vi "CIVITA_DMARS_conv_PXI(SubVI).vi"(8 "Initial Euler Angles [rad]":cluster{"phi":dbl, "theta":dbl, "psi":dbl}={"phi"=0.766, "theta"=0.643, "psi"=0.0}, 10 "SIM_start":bool, 11 "Civitanav readings [deg]":sgl[](array[numeric])) -> (2 "psi [deg]":dbl, 3 "Euler Angles [rad]":cluster{"phi":dbl, "theta":dbl, "psi":dbl}, 5 "theta [deg]":dbl, 7 "phi [deg]":dbl)   [LabVIEW 2017]
uses:
  <vilib>/Analysis/coordinate.llb/Euler Rotation Order.ctl
  <vilib>/Analysis/baseanly.llb/Real A x B.vi
  <vilib>/Analysis/Matrix/Numeric/Conversions/Array To Matrix - RA2.vi
  <vilib>/Analysis/Matrix/Numeric/Conversions/Matrix To Array - RM.vi
  <vilib>/Analysis/NI_AALPro.lvlib
  <vilib>/Analysis/NI_AALBase.lvlib
  <vilib>/Analysis/Matrix/NI_Matrix.lvlib
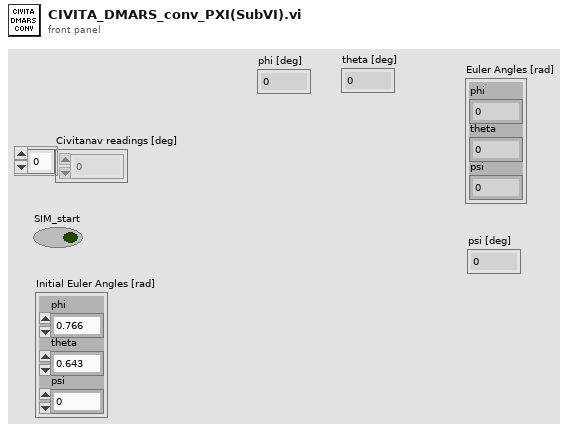
[diagram p1: front panel]
types:
  T1 = typedef "NI_AALPro.lvlib/Euler Rotation Order.ctl" = u16
  T2 = typedef "NI_Matrix.lvlib/RealMatrix.ctl" = dbl[][]
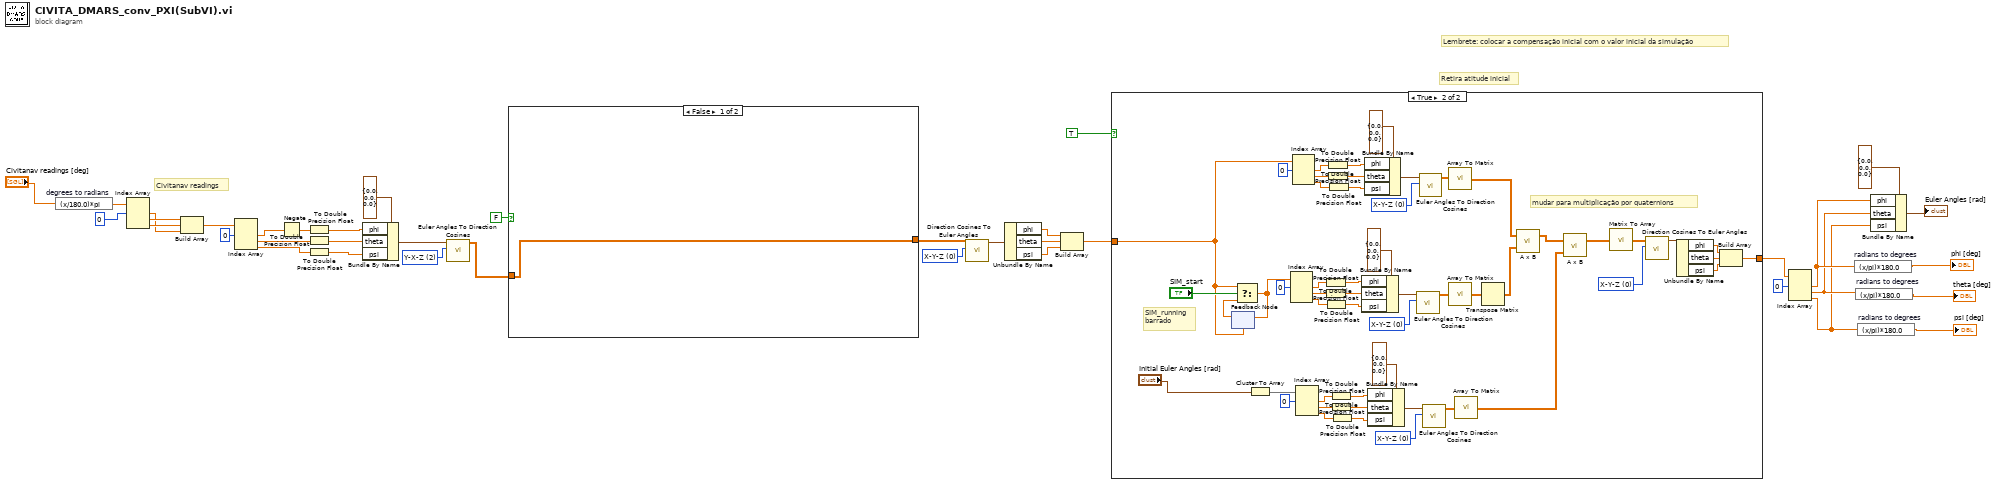
[diagram p0: block diagram]
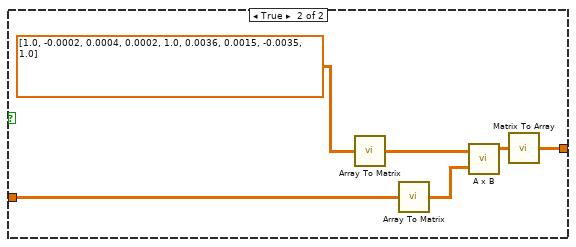
[diagram p3: hidden frame]
diagram:
  w36 = T1 0 items=["X-Y-Z", "X-Z-Y", "Y-X-Z", "Y-Z-X", "Z-X-Y", "Z-Y-X", "X-Y-X", "X-Z-X", "Y-X-Y", "Y-Z-Y", "Z-X-Z", "Z-Y-Z"] ("rotation order")
  w37 = T1 2 items=["X-Y-Z", "X-Z-Y", "Y-X-Z", "Y-Z-X", "Z-X-Y", "Z-Y-X", "X-Y-X", "X-Z-X", "Y-X-Y", "Y-Z-Y", "Z-X-Z", "Z-Y-Z"] ("rotation order")
  # "Lembrete: colocar a compensação inicial com o valor inicial da simulação"
  # "Retira atitude inicial"
  # "Civitanav readings"
  n1 = expression code="(x/180.0)*pi" "degrees to radians"("Civitanav readings [deg]") -> (w31:sgl[])
  n2 = Index Array(array=w31, index #1=0 ("index")) -> (element #1=w27:sgl, element #2=w29:sgl, element #3=w28:sgl)  [unwired: 2 in]
  n3 = Build Array(w29, w28, w27) -> (w17:sgl[])
  n4 = Index Array(array=w17, index #1=0 ("index")) -> (element #1=w23:sgl, element #2=w21:sgl, element #3=w20:sgl)  [unwired: 2 in]
  n5 = Negate(x=w23) -> (-x=w22:sgl)
  n6 = To Double Precision Float(number=w22) -> (double precision float=w3:dbl)
  n7 = To Double Precision Float(number=w21) -> (double precision float=w1:dbl)
  n8 = To Double Precision Float(number=w20) -> (double precision float=w2:dbl)
  n9 = Bundle By Name(cluster=cluster{"phi":dbl, "theta":dbl, "psi":dbl} {"phi"=0.0, "theta"=0.0, "psi"=0.0} ("Euler Angles"), "phi"=w3, "theta"=w1, "psi"=w2) -> (w34:cluster{"phi":dbl, "theta":dbl, "psi":dbl})
  n10 = call <vilib>:"Euler Angles To Direction Cosines.vi"("rotation order"=w37, "Euler Angles"=w34) -> ("Direction Cosines"=w4:dbl[][])  [unwired: 8 in, 1 out]
  n11 = case shown="False" FALSE {
    tunnel: [w39 w42] -> w19
    tunnel: w4 -> [w39 w40]
    frame False {
    }
    frame True {
      n12 = call-poly <vilib>:"Array To Matrix.vi"("Real 2D Array"=dbl[][] [[1.0, -0.0002, 0.0004], [0.0002, 1.0, 0.0036], [0.0015, -0.0035, 1.0]]) -> ("Real Matrix"=w44:T2)
      n13 = call-poly <vilib>:"Array To Matrix.vi"("Real 2D Array"=w40) -> ("Real Matrix"=w43:T2)
      n14 = call-poly <vilib>:"A x B.vi"("B"=w43, "A"=w44) -> ("A x B"=w45:T2)  [unwired: 1 out]
      n15 = call-poly <vilib>:"Matrix To Array.vi"("Real Matrix"=w45) -> ("Real 2D Array"=w42:dbl[][])
    }
  }
  n16 = call <vilib>:"Direction Cosines To Euler Angles.vi"("rotation order"=w36, "Direction Cosines"=w19) -> ("Euler Angles"=w38:cluster{"phi":dbl, "theta":dbl, "psi":dbl})  [unwired: 8 in, 1 out]
  n17 = Unbundle By Name(w38) -> ("phi"=w15:dbl, "theta"=w14:dbl, "psi"=w13:dbl)
  n18 = Build Array(w15, w14, w13) -> (w12:dbl[])
  n19 = case shown="True" TRUE {
    tunnel: w12 -> [w46 w67]
    tunnel: [w46 w65] -> w11
    frame False {
    }
    frame True {
      w56 = T1 0 items=["X-Y-Z", "X-Z-Y", "Y-X-Z", "Y-Z-X", "Z-X-Y", "Z-Y-X", "X-Y-X", "X-Z-X", "Y-X-Y", "Y-Z-Y", "Z-X-Z", "Z-Y-Z"] ("rotation order")
      w72 = T1 0 items=["X-Y-Z", "X-Z-Y", "Y-X-Z", "Y-Z-X", "Z-X-Y", "Z-Y-X", "X-Y-X", "X-Z-X", "Y-X-Y", "Y-Z-Y", "Z-X-Z", "Z-Y-Z"] ("rotation order")
      w80 = T1 0 items=["X-Y-Z", "X-Z-Y", "Y-X-Z", "Y-Z-X", "Z-X-Y", "Z-Y-X", "X-Y-X", "X-Z-X", "Y-X-Y", "Y-Z-Y", "Z-X-Z", "Z-Y-Z"] ("rotation order")
      w93 = T1 0 items=["X-Y-Z", "X-Z-Y", "Y-X-Z", "Y-Z-X", "Z-X-Y", "Z-Y-X", "X-Y-X", "X-Z-X", "Y-X-Y", "Y-Z-Y", "Z-X-Z", "Z-Y-Z"] ("rotation order")
      # "mudar para multiplicação por quaternions"
      # "SIM_running\nbarrado"
      n20 = feedback #1(w67) -> (w97:dbl[])
      n21 = Select(t=w67, s="SIM_start", f=w97) -> (s? t:f=w66:dbl[])
      n22 = feedback-in #1(w66) -> ()
      n23 = Cluster To Array(cluster="Initial Euler Angles [rad]") -> (array=w48:dbl[])
      n24 = Index Array(array=w66, index #1=0 ("index")) -> (element #1=w81:dbl, element #2=w82:dbl, element #3=w83:dbl)  [unwired: 2 in]
      n25 = Index Array(array=w67, index #1=0 ("index")) -> (element #1=w92:dbl, element #2=w91:dbl, element #3=w90:dbl)  [unwired: 2 in]
      n26 = Index Array(array=w48, index #1=0 ("index")) -> (element #1=w57:dbl, element #2=w58:dbl, element #3=w59:dbl)  [unwired: 2 in]
      n27 = To Double Precision Float(number=w81) -> (double precision float=w84:dbl)
      n28 = To Double Precision Float(number=w82) -> (double precision float=w85:dbl)
      n29 = To Double Precision Float(number=w83) -> (double precision float=w86:dbl)
      n30 = To Double Precision Float(number=w92) -> (double precision float=w89:dbl)
      n31 = To Double Precision Float(number=w91) -> (double precision float=w88:dbl)
      n32 = To Double Precision Float(number=w90) -> (double precision float=w87:dbl)
      n33 = To Double Precision Float(number=w57) -> (double precision float=w60:dbl)
      n34 = To Double Precision Float(number=w58) -> (double precision float=w61:dbl)
      n35 = To Double Precision Float(number=w59) -> (double precision float=w62:dbl)
      n36 = Bundle By Name(cluster=cluster{"phi":dbl, "theta":dbl, "psi":dbl} {"phi"=0.0, "theta"=0.0, "psi"=0.0} ("Euler Angles"), "phi"=w84, "theta"=w85, "psi"=w86) -> (w79:cluster{"phi":dbl, "theta":dbl, "psi":dbl})
      n37 = Bundle By Name(cluster=cluster{"phi":dbl, "theta":dbl, "psi":dbl} {"phi"=0.0, "theta"=0.0, "psi"=0.0} ("Euler Angles"), "phi"=w89, "theta"=w88, "psi"=w87) -> (w94:cluster{"phi":dbl, "theta":dbl, "psi":dbl})
      n38 = Bundle By Name(cluster=cluster{"phi":dbl, "theta":dbl, "psi":dbl} {"phi"=0.0, "theta"=0.0, "psi"=0.0} ("Euler Angles"), "phi"=w60, "theta"=w61, "psi"=w62) -> (w55:cluster{"phi":dbl, "theta":dbl, "psi":dbl})
      n39 = call <vilib>:"Euler Angles To Direction Cosines.vi"("rotation order"=w80, "Euler Angles"=w79) -> ("Direction Cosines"=w75:dbl[][])  [unwired: 8 in, 1 out]
      n40 = call <vilib>:"Euler Angles To Direction Cosines.vi"("rotation order"=w93, "Euler Angles"=w94) -> ("Direction Cosines"=w76:dbl[][])  [unwired: 8 in, 1 out]
      n41 = call <vilib>:"Euler Angles To Direction Cosines.vi"("rotation order"=w56, "Euler Angles"=w55) -> ("Direction Cosines"=w53:dbl[][])  [unwired: 8 in, 1 out]
      n42 = call-poly <vilib>:"Array To Matrix.vi"("Real 2D Array"=w76) -> ("Real Matrix"=w63:T2)
      n43 = call-poly <vilib>:"Array To Matrix.vi"("Real 2D Array"=w75) -> ("Real Matrix"=w74:T2)
      n44 = call-poly <vilib>:"Array To Matrix.vi"("Real 2D Array"=w53) -> ("Real Matrix"=w51:T2)
      n45 = Transpose Matrix(1:w74) -> (0:w64:T2)
      n46 = call-poly <vilib>:"A x B.vi"("B"=w64, "A"=w63) -> ("A x B"=w50:T2)  [unwired: 1 out]
      n47 = call-poly <vilib>:"A x B.vi"("B"=w51, "A"=w50) -> ("A x B"=w49:T2)  [unwired: 1 out]
      n48 = call-poly <vilib>:"Matrix To Array.vi"("Real Matrix"=w49) -> ("Real 2D Array"=w73:dbl[][])
      n49 = call <vilib>:"Direction Cosines To Euler Angles.vi"("rotation order"=w72, "Direction Cosines"=w73) -> ("Euler Angles"=w71:cluster{"phi":dbl, "theta":dbl, "psi":dbl})  [unwired: 8 in, 1 out]
      n50 = Unbundle By Name(w71) -> ("phi"=w70:dbl, "theta"=w69:dbl, "psi"=w68:dbl)
      n51 = Build Array(w70, w69, w68) -> (w65:dbl[])
    }
  }
  n52 = Index Array(array=w11, index #1=0 ("index")) -> (element #1=w8:dbl, element #2=w7:dbl, element #3=w6:dbl)  [unwired: 2 in]
  n53 = expression code="(x/pi)*180.0" "radians to degrees"(w8) -> (→"phi [deg]":dbl)
  n54 = expression code="(x/pi)*180.0" "radians to degrees"(w7) -> (→"theta [deg]":dbl)
  n55 = expression code="(x/pi)*180.0" "radians to degrees"(w6) -> (→"psi [deg]":dbl)
  n56 = Bundle By Name(cluster=cluster{"phi":dbl, "theta":dbl, "psi":dbl} {"phi"=0.0, "theta"=0.0, "psi"=0.0} ("Euler Angles 2"), "phi"=w8, "theta"=w7, "psi"=w6) -> (→"Euler Angles [rad]":cluster{"phi":dbl, "theta":dbl, "psi":dbl})
